vi "myFreqParamGen.vi"(0 "freqs":i32[](array[numeric])=[10, 14, 19, 27, 37, 51, 71, 99, 140, 190, 260, 360, 510, 700, 970, 1400, 1900, 2600, 3600, 5000], 1 "响应测试选项":u8(ring)=3 items=["仅测量信号", "单相扫频", "三相同步系扫频", "三相正负序扫频"], 2 "频率分辨率上限\nf_tick_ref":u32=10 min=1 max=100000, 3 "测量周期数 n":u32=2 min=1 max=10, 5 "freqs group":i32[][](array[numeric]), 7 "freqs index":i32[][](array[numeric]), 9 "freqs ind group":i32[][](array[numeric]), 11 "基波频率 f_fun":u32=50 min=1 max=100000, 12 "sample_0":u64=1000000, 13 "timebase_0":u32=127) -> (4 "扫频点取值报告":string, 6 "扫频点密度及其采样时长预览":cluster{"freqs":i32[], "freqs":dbl[]}[](graph), 14 "最大同时使用内存(kS)":u64 caption="单频点最大使用内存(kS)")   [LabVIEW 2024]
doc: "根据频率组，生成它在采样中需要的采样量与分辨率。\n同时输出各频率对应的，在FFT结果中的索引。"
panel:
  out "fft_index":i32[][](array[numeric])
  out "n_tbase":u32[](array[numeric])
  out "n_samp":u64[](array[numeric])
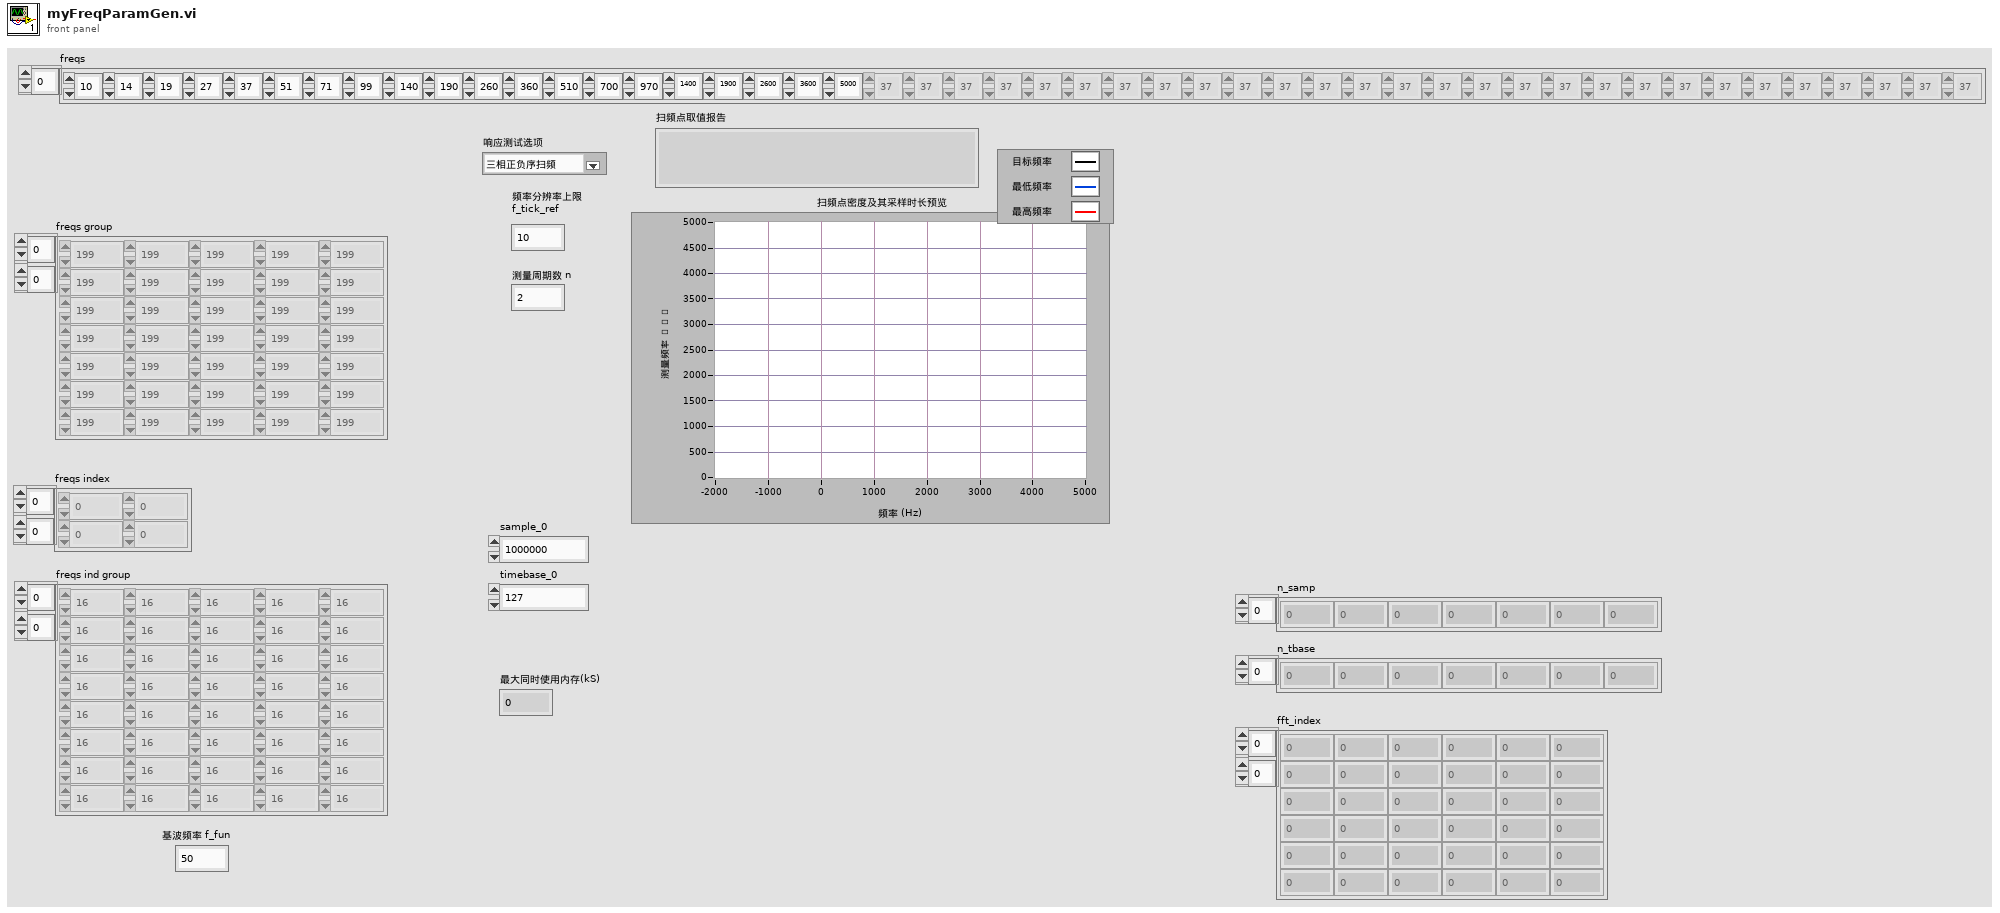
[diagram p1: front panel]
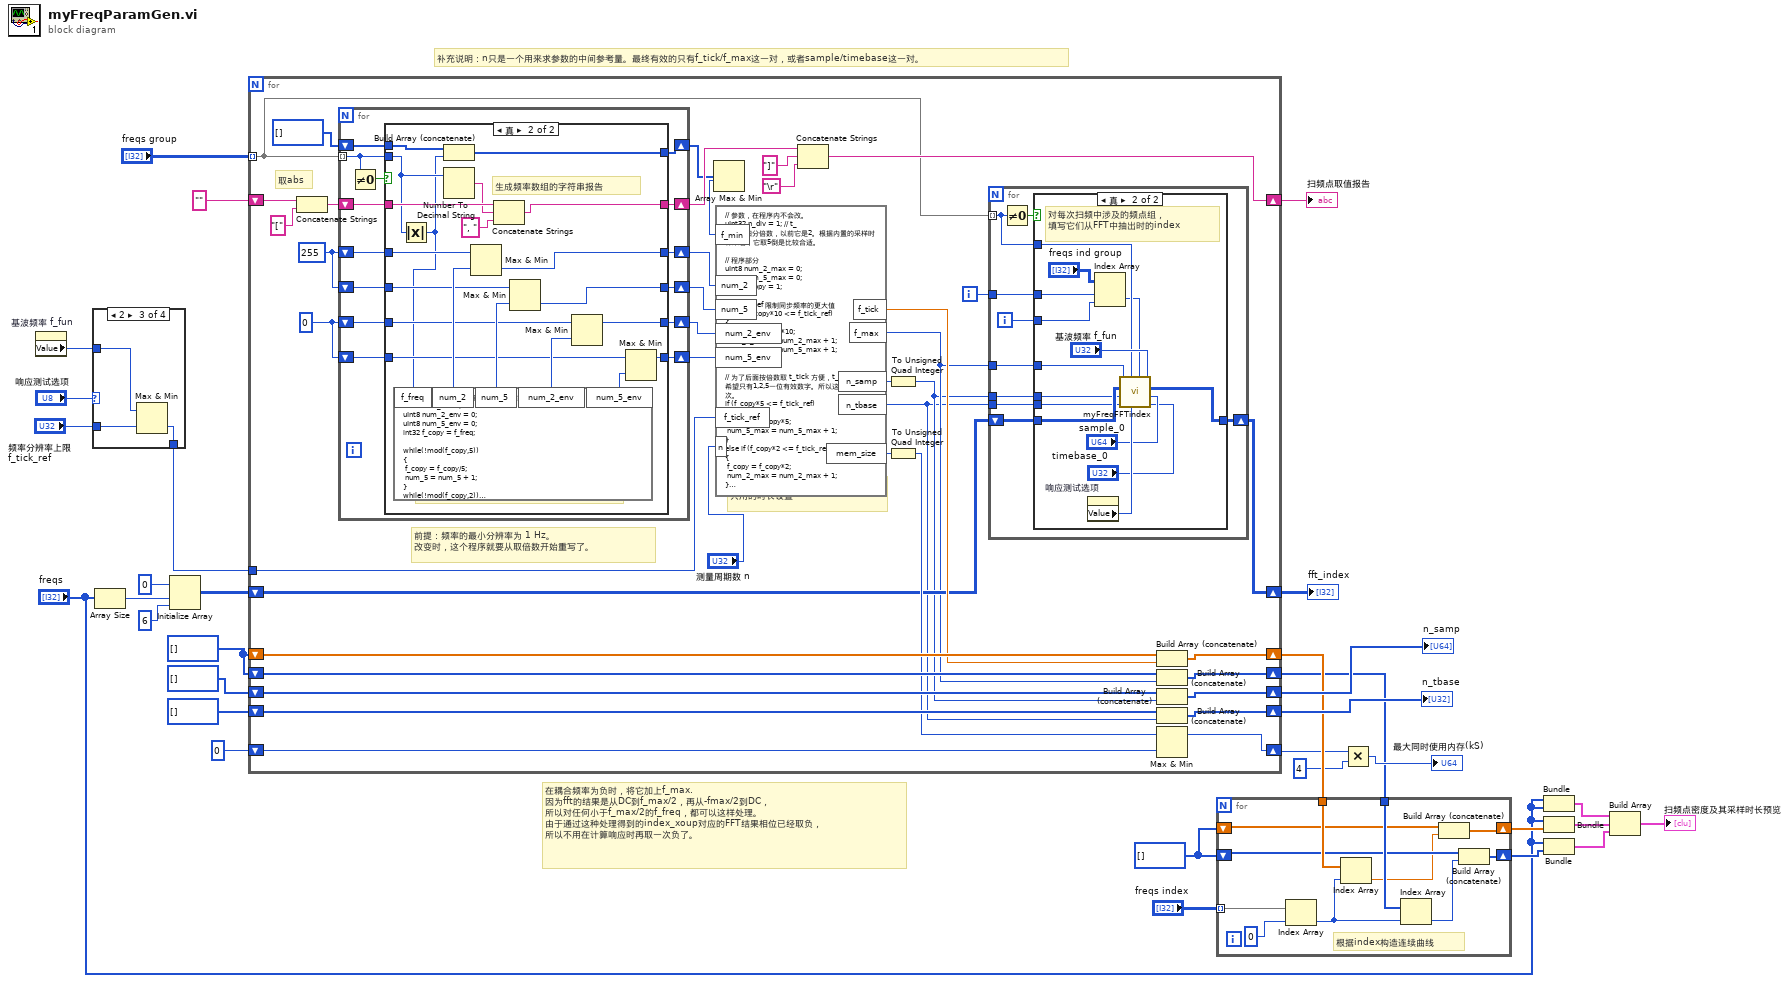
[diagram p0: block diagram]
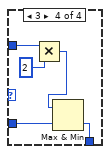
[diagram p4: hidden frame]
diagram:
  w23 = i32[] []
  w30 = i32[] []
  # "在耦合频率为负时，将它加上f_max.\n因为fft的结果是从DC到f_max/2，再从-fmax/2到DC，\n所以对任何小于f_max/2的f_freq，都可以这样处理。\n由于通过这种处理得到的index_xoup对应的FFT结果相位已经取负，\n所以不用在计算响应时再取一次负了。"
  # "补充说明：n只是一个用来求参数的中间参考量。最终有效的只有f_tick/f_max这一对，或者sample/timebase这一对。"
  n1 = property on="基波频率 f_fun" class="DigNum (严格)"() -> ("Value"=w2:u32)  [unwired: 2 in, 2 out]
  n2 = case shown="2" "响应测试选项" {
    tunnel: "频率分辨率上限\nf_tick_ref" -> [w33 w34 w37 w41]
    tunnel: [w33 w34 w36 w42] -> w13
    tunnel: w2 -> [_ _ w35 w40]
    frame 0, Default {
    }
    frame 1 {
    }
    frame 2 {
      n3 = Max & Min(x=w35, y=w37) -> (min(x,y)=w36:u32)  [unwired: 1 out]
    }
    frame 3 {
      n4 = Multiply(x=w40, y=u32 2) -> (x*y=w38:u32)
      n5 = Max & Min(x=w38, y=w41) -> (min(x,y)=w42:u32)  [unwired: 1 out]
    }
  }
  n6 = Array Size(array="freqs") -> (size(s)=w9:i32)
  n7 = Initialize Array(0 ("维数大小"), w9, 6 ("维数大小")) -> (w8:i32[][])
  n8 = for {
    tunnel: "freqs group" -> [w43] mode=indexing
    shift-right: [w76] -> w31
    shift-left: "" -> [w80]
    shift-right: [w64] -> w24
    shift-left: w30 -> [w69]
    shift-right: [w65] -> w1
    shift-left: w30 -> [w61]
    shift-right: [w66] -> w26
    shift-left: u64[] [] -> [w62]
    shift-right: [w67] -> w25
    shift-left: u32[] [] -> [w63]
    shift-right: [w71] -> w4
    shift-left: u64 0 -> [w70]
    tunnel: w13 -> [w51]
    shift-right: [w47] -> w6
    shift-left: w8 -> [w49]
    i -> [w50]
    w55 = u8 0
    w73 = u8 255
    # "取abs"
    # "前提：频率的最小分辨率为 1 Hz。\n改变时，这个程序就要从取倍数开始重写了。"
    # "对这一行，确定该注入周期，\n共用的时长设置"
    n9 = Concatenate Strings(w80, "[") -> (w79:string)
    n10 = for {
      tunnel: w43 -> [w117] mode=indexing
      shift-right: [w116] -> w72
      shift-left: i32[] [] -> [w119]
      shift-right: [w115] -> w77
      shift-left: w79 -> [w114]
      shift-right: [w111] -> w57
      shift-left: w73 -> [w113]
      shift-right: [w110] -> w56
      shift-left: w73 -> [w112]
      shift-right: [w108] -> w54
      shift-left: w55 -> [w106]
      shift-right: [w109] -> w53
      shift-left: w55 -> [w107]
      n11 = Not Equal To 0?(x=w117) -> (x != 0?=w118:bool)
      n12 = case shown="真" w118 {
        tunnel: w119 -> [w125 w145]
        tunnel: w117 -> [_ w127]
        tunnel: [w125 w144] -> w116
        tunnel: [w124 w142] -> w115
        tunnel: w114 -> [w124 w141]
        tunnel: [w122 w139] -> w110
        tunnel: [w123 w138] -> w111
        tunnel: w113 -> [w123 w135]
        tunnel: w112 -> [w122 w134]
        tunnel: [w120 w133] -> w109
        tunnel: [w121 w132] -> w108
        tunnel: w107 -> [w120 w129]
        tunnel: w106 -> [w121 w128]
        frame False {
        }
        frame True {
          # "生成频率数组的字符串报告"
          # "对每一行频率组，\n求当前所有f_freq相对1Hz的，\nt相对1ns的2的数量，5的数量\n在该方法下求最大公因数和最小公倍数"
          n13 = Absolute Value(x=w127) -> (abs(x)=w126:i32)
          n14 = formula code="uInt8 num_2 = 0;\t// 输出，寄存构造数组\nuInt8 num_5 = 0;\nuInt8 num_2_env = 0;\nuInt8 num_5_env = 0;\nint32 f_copy = f_freq;\n\nwhile(!mod(f_copy,5))\n{\n\tf_copy = f_copy/5;\n\tnum_5 = num_5 + 1;\n}\nwhile(!mod(f_copy,2))\n{\n\tf_copy = f_copy/2;\n\tnum_2 = num_2 + 1;\n}\n\n// 计算：包络频率\nf_copy = 1;\nwhile (f_copy*10 <= f_freq)\n{\n\tnum_2_env = num_2_env+1;\n\tnum_5_env = num_5_env+1;\n\tf_copy = f_copy*10;\n}\nif (f_copy*2 >= f_freq)\n{\n\tnum_2_env = num_2_env+1;\n\tf_copy = f_copy*2;\n}\nelse if (f_copy*5 >= f_freq)\n{\n\tnum_5_env = num_5_env+1;\n\tf_copy = f_copy*5;\n}\nelse\n{\n\tnum_2_env = num_2_env+1;\n\tnum_5_env = num_5_env+1;\n\tf_copy = f_copy*10;\n}"("f_freq"=w126) -> ("num_2"=w136:u8, "num_5"=w137:u8, "num_2_env"=w130:u8, "num_5_env"=w131:u8)
          n15 = Build Array (concatenate)(w145, w126) -> (w144:i32[])
          n16 = Number To Decimal String(number=w127) -> (decimal integer string=w140:string)  [unwired: 1 in]
          n17 = Max & Min(x=w135, y=w136) -> (min(x,y)=w138:u8)  [unwired: 1 out]
          n18 = Concatenate Strings(w141, w140, ", ") -> (w142:string)
          n19 = Max & Min(x=w134, y=w137) -> (min(x,y)=w139:u8)  [unwired: 1 out]
          n20 = Max & Min(x=w128, y=w130) -> (max(x,y)=w132:u8)  [unwired: 1 out]
          n21 = Max & Min(x=w129, y=w131) -> (max(x,y)=w133:u8)  [unwired: 1 out]
        }
      }
    }
    n22 = Array Max & Min(array=w72) -> (min value=w52:i32)  [unwired: 3 out]
    n23 = formula code="// 参数，在程序内不会改。\nuInt32 n_div = 1;\t// t_tick的细分倍数，以前它是2。根据内置的采样时钟来看，它取5倒是比较合适。\n\n// 程序部分\nuInt8 num_2_max = 0;\nuInt8 num_5_max = 0;\nint32 f_copy = 1;\n\n// f_tick_ref 限制同步频率的更大值\nwhile (f_copy*10 <= f_tick_ref)\n{\n\tf_copy = f_copy*10;\n\tnum_2_max = num_2_max + 1;\n\tnum_5_max = num_5_max + 1;\n}\n\n// 为了后面按倍数取 t_tick 方便，t_max 希望只有1,2,5一位有效数字。所以这里只判断一次。\nif (f_copy*5 <= f_tick_ref)\n{\n\tf_copy = f_copy*5;\n\tnum_5_max = num_5_max + 1;\n}\nelse if (f_copy*2 <= f_tick_ref)\n{\n\tf_copy = f_copy*2;\n\tnum_2_max = num_2_max + 1;\n}\n\n// 以 f_tick_ref 为最大值寻找同步频率\nuInt8 num_2_last = min(num_2, num_2_max);\nuInt8 num_5_last = min(num_5, num_5_max);\n\n// 将两个因数次数的差值控制在 1 之内\nif (num_2_last > num_5_last)\n{\n\tnum_2_last = num_5_last + 1;\n}\nelse if (num_5_last > num_2_last)\n{\n\tnum_5_last = num_2_last + 1;\n}\n\n// 计算：在要求范围内的采样总时长\nint32 f_tick_int = pow(2,num_2_last)*pow(5,num_5_last);\n// 修正：过大同步频率的收缩\nif (f_tick_int == f_min)\n{\n\tif (num_5_last >= num_2_last & num_5_last >= 1)\n\t{\n\t\tf_tick_int = f_tick_int/5;\n\t\t}\n\telse if (num_2_last > num_5_last & num_2_last >= 1)\n\t{\n\t\tf_tick_int = f_tick_int/2;\n\t\t}\n}\n\n// 计算：细分最小时长\nint32 f_max = min(n_div * max(1e3 * f_tick_int,pow(2,num_2_env)*pow(5,num_5_env)),5e6);\t// 它一定只有一位有效数字。因此 n_tbase 一定是整数。\n// 修正：最小时长取整（应该不会发生这种情况）\nwhile(mod(125e6,f_max))\n{\n\tf_max = f_max/2;\n}\n\n// 计算：后续参数\nuInt32 n_samp = f_max/f_tick_int;\t// 示波器的sample数\nuInt32 n_tbase = (1e9/f_max+16)/8;\t// 示波器的timebase数\n\n// 修正：采样周期补正\nn_samp = n_samp * n;\nuInt32 mem_size = 4*n_samp/1e3;\n\n// 输出：整数变浮点数\nfloat f_tick = f_tick_int/n;"("num_2"=w57, "num_5"=w56, "f_tick_ref"=w51, "n"="测量周期数 n", "num_2_env"=w54, "num_5_env"=w53, "f_min"=w52) -> ("f_tick"=w68:dbl, "f_max"=w46:i32, "n_samp"=w60:u32, "n_tbase"=w44:u32, "mem_size"=w58:u32)
    n24 = Concatenate Strings(w77, "]", "\r") -> (w76:string)
    n25 = To Unsigned Quad Integer(1:w60) -> (0:w45:u64)
    n26 = To Unsigned Quad Integer(1:w58) -> (0:w59:u64)
    n27 = for {
      tunnel: w50 -> [w89]
      tunnel: w43 -> [w87] mode=indexing
      shift-right: [w85] -> w47
      shift-left: w49 -> [w86]
      tunnel: w46 -> [w84]
      tunnel: w45 -> [w83]
      tunnel: w44 -> [w82]
      i -> [w88]
      n28 = Not Equal To 0?(x=w87) -> (x != 0?=w90:bool)
      n29 = case shown="真" w90 {
        tunnel: w89 -> [_ w104]
        tunnel: w88 -> [_ w103]
        tunnel: w87 -> [_ w95]
        tunnel: w86 -> [w91 w102]
        tunnel: [w91 w101] -> w85
        tunnel: w84 -> [_ w96]
        tunnel: w83 -> [_ w93]
        tunnel: w82 -> [_ w92]
        frame False {
        }
        frame True {
          # "对每次扫频中涉及的频点组，\n填写它们从FFT中抽出时的index"
          n30 = property on="响应测试选项" class="Ring (严格)"() -> ("Value"=w99:u8)  [unwired: 2 in, 2 out]
          n31 = Index Array(array="freqs ind group", index (row)=w104, index (col)=w103) -> (element=w94:i32)
          n32 = call "myFreqFFTindex.vi"("n_timebase_0"="timebase_0", "n_sample_0"="sample_0", "f_fun"="基波频率 f_fun", "freqs_index"=w94, "sweep_mode"=w99, "f_freq"=w95, "n_timebase_f"=w92, "n_sample_f"=w93, "fft_index_in"=w102, "f_max"=w96) -> ("fft_index_out"=w101:i32[][])  [unwired: 1 in]
        }
      }
    }
    n33 = Build Array (concatenate)(w69, w68) -> (w64:dbl[])
    n34 = Build Array (concatenate)(w61, w46) -> (w65:i32[])
    n35 = Build Array (concatenate)(w62, w45) -> (w66:u64[])
    n36 = Build Array (concatenate)(w63, w44) -> (w67:u32[])
    n37 = Max & Min(x=w59, y=w70) -> (max(x,y)=w71:u64)  [unwired: 1 out]
  }
  "扫频点取值报告" <- w31
  "n_samp" <- w26
  "n_tbase" <- w25
  "fft_index" <- w6
  n38 = for {
    tunnel: "freqs index" -> [w156] mode=indexing
    tunnel: w24 -> [w154]
    tunnel: w1 -> [w153]
    shift-right: [w148] -> w17
    shift-left: w23 -> [w147]
    shift-right: [w151] -> w21
    shift-left: w23 -> [w150]
    # "根据index构造连续曲线"
    n39 = Index Array(array=w156, index=0) -> (element=w152:i32)
    n40 = Index Array(array=w154, index=w152) -> (element=w146:dbl)
    n41 = Index Array(array=w153, index=w152) -> (element=w149:i32)
    n42 = Build Array (concatenate)(w147, w146) -> (w148:dbl[])
    n43 = Build Array (concatenate)(w150, w149) -> (w151:i32[])
  }
  n44 = Multiply(x=w4, y=u64 4) -> (x*y=→"最大同时使用内存(kS)":u64)
  n45 = Bundle("freqs"="freqs", "freqs"="freqs") -> (w20:cluster{"freqs":i32[], "freqs":i32[]})  [unwired: 1 in]
  n46 = Bundle("freqs"="freqs", w17) -> (w19:cluster{"freqs":i32[], dbl[]})  [unwired: 1 in]
  n47 = Bundle("freqs"="freqs", w21) -> (w18:cluster{"freqs":i32[], i32[]})  [unwired: 1 in]
  n48 = Build Array(w20, w19, w18) -> (→"扫频点密度及其采样时长预览":cluster{"freqs":i32[], "freqs":dbl[]}[])
